vi "2 PolarPlot.vi"(1 "Apparent Wind\nSpeed":T2, 2 "Apparent Wind\nDirection (º)":T3, 3 "Boat Angle":dbl) -> (0 "Velocity":dbl)   [LabVIEW 2011]
uses:
  2 Typedefs/apparent wind direction.ctl
  2 Typedefs/apparent wind speed.ctl
  2 Classes/LinearInterpolation/AngleValuePair.ctl
  2 Classes/LinearInterpolation/LinearInterpolation.lvclass
  2 Globals/2 TuningConstants.vi
panel:
  out "Array":T1[](array[typedef])
  out "Irons Range":dbl=40.0 step=0.1
  in  "Angle-Value Pairs":T1[](array[typedef])=[{"Angle (deg)"=0.0, "Value"=0.0}, {"Angle (deg)"=44.9, "Value"=0.0}, {"Angle (deg)"=45.0, "Value"=0.85}, {"Angle (deg)"=90.0, "Value"=1.0}, {"Angle (deg)"=160.0, "Value"=1.0}, {"Angle (deg)"=180.0, "Value"=0.9}, {"Angle (deg)"=200.0, "Value"=1.0}, {"Angle (deg)"=270.0, "Value"=1.0}, {"Angle (deg)"=315.0, "Value"=0.85}, {"Angle (deg)"=315.136, "Value"=0.0}, {"Angle (deg)"=360.0, "Value"=0.0}]
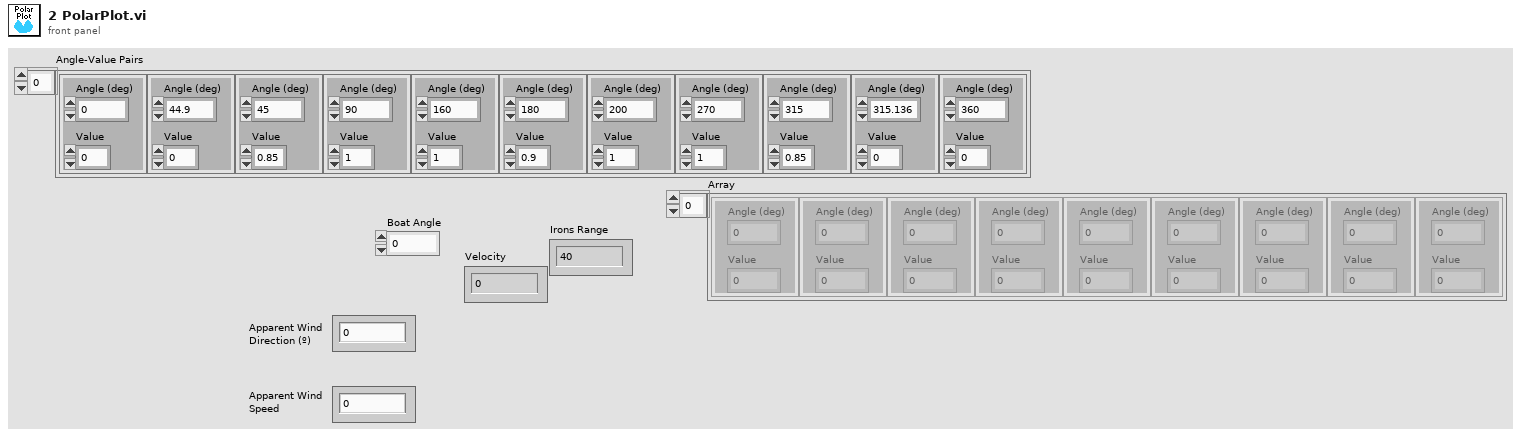
[diagram p1: front panel]
types:
  T1 = typedef "AngleValuePair.ctl" = cluster{"Angle (deg)":dbl, "Value":dbl}
  T2 = typedef "apparent wind speed.ctl" = dbl
  T3 = typedef "apparent wind direction.ctl" = dbl
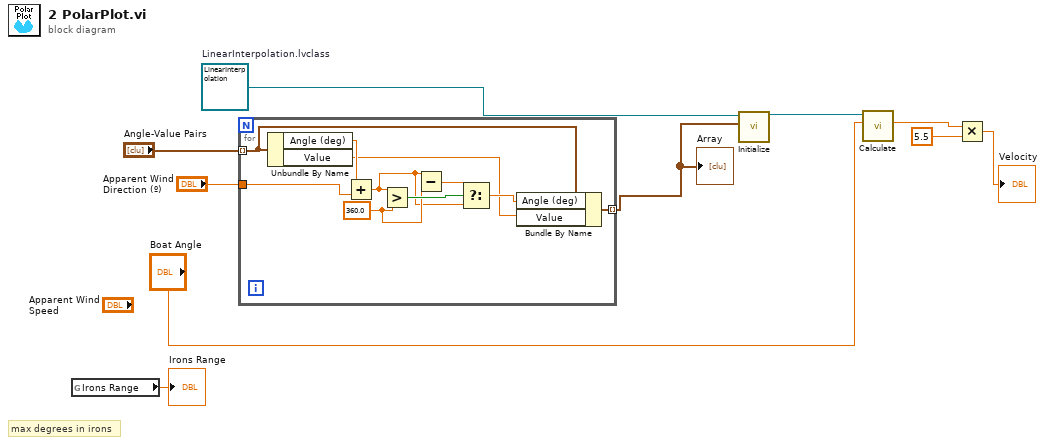
[diagram p0: block diagram]
diagram:
  w10 = refnum<class "LinearInterpolation.lvclass"> refnum  # LinearInterpolation.lvclass
  # "max degrees in irons"
  n1 = global read "2 TuningConstants.vi" "Irons Range"() -> (→"Irons Range":dbl)
  n2 = for {
    tunnel: "Angle-Value Pairs" -> [w14] mode=indexing
    tunnel: "Apparent Wind\nDirection (º)" -> [w20]
    tunnel: [w12] -> w1 mode=indexing
    w17 = 360.0 ("y")
    n3 = Unbundle By Name(w14) -> ("Angle (deg)"=w19:dbl, "Value"=w11:dbl)
    n4 = Add(x=w19, y=w20) -> (x+y=w15:T3)
    n5 = Greater?(x=w15, y=w17) -> (0:w18:bool)
    n6 = Subtract(x=w15, y=w17) -> (x-y=w16:T3)
    n7 = Select(t=w16, s=w18, f=w15) -> (s? t:f=w13:T3)
    n8 = Bundle By Name(cluster=w14, "Angle (deg)"=w13, "Value"=w11) -> (w12:T1)
  }
  "Array" <- w1
  n9 = call "Initialize.vi"("Angle-Value Pairs"=w1, "LinearInterpolation in"=w10) -> ("LinearInterpolation out"=w5:refnum<class "LinearInterpolation.lvclass">)  [unwired: 8 in, 1 out]
  n10 = call-dynamic "Calculate.vi"("X (degrees)"="Boat Angle", "AngleFunction in"=w5) -> ("AngleFunction(X)"=w8:dbl)  [unwired: 7 in, 2 out]
  n11 = Multiply(x=w8, y=5.5) -> (x*y=→"Velocity":dbl)
